vi "model thread map--fgv.vi"(2 "operation":enum16{"Reset", "Insert", "Remove", "find"}(ring), 5 "model name in":string, 7 "model number in":i32, 9 "thread number In":i32, 11 "error in (no error)":errorcluster) -> (4 "Map":map{string, i32}(c390), 6 "model name out":string, 8 "model number out":i32, 10 "thread number out":i32, 15 "error out":errorcluster)   [LabVIEW 2022 SP3]
uses:
  <vilib>/Utility/error.llb/Error Cluster From Error Code.vi
  <vilib>/ErrorRing/Error Ring.xnode
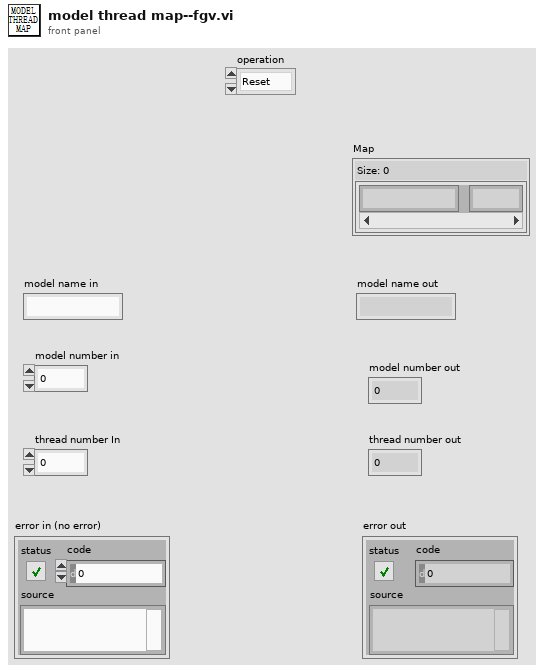
[diagram p1: front panel]
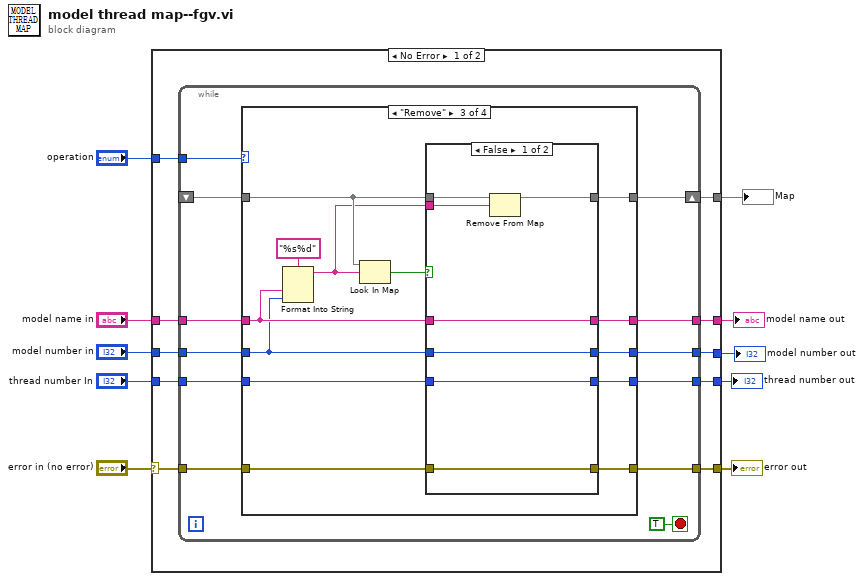
[diagram p0: block diagram]
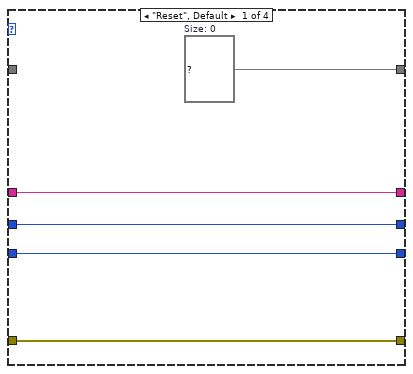
[diagram p2: hidden frame]
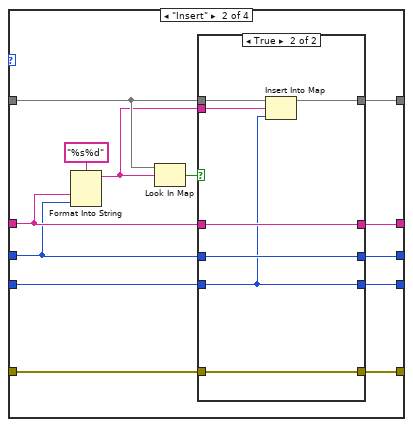
[diagram p3: hidden frame]
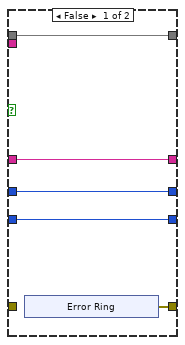
[diagram p4: hidden frame]
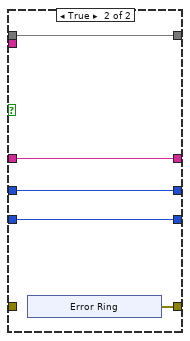
[diagram p5: hidden frame]
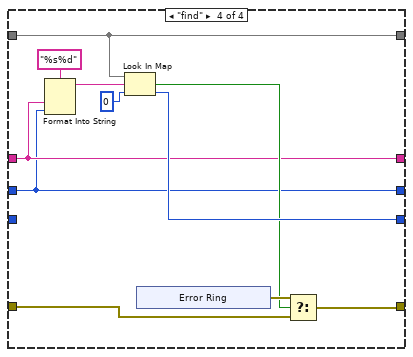
[diagram p6: hidden frame]
diagram:
  n1 = case shown="No Error" "error in (no error)" {
    selector: "error in (no error)" -> [w15 w117]
    tunnel: "operation" -> [w20 _]
    tunnel: "model name in" -> [w19 w116]
    tunnel: "model number in" -> [w18 w115]
    tunnel: [w16 w117] -> w6
    tunnel: "thread number In" -> [w17 w114]
    tunnel: [w14 w114] -> w4
    tunnel: [w13 _] -> w3
    tunnel: [w12 w116] -> w2
    tunnel: [w11 w115] -> w1
    frame No Error {
      n2 = while {
        shift-right: [w30] -> w13
        shift-left: _ -> [w29]
        tunnel: w20 -> [w32]
        tunnel: w19 -> [w28]
        tunnel: w18 -> [w27]
        tunnel: w17 -> [w26]
        tunnel: [w25] -> w16
        tunnel: w15 -> [w24]
        tunnel: [w23] -> w14
        tunnel: [w22] -> w12
        tunnel: [w21] -> w11
        stop <- TRUE stop-if-true
        n3 = case shown="\"Remove\"" w32 {
          tunnel: [w37 w47 w77 w106] -> w30
          tunnel: w29 -> [_ w48 w78 w106]
          tunnel: w28 -> [w35 w42 w73 w99]
          tunnel: w27 -> [w34 w40 w72 w98]
          tunnel: w26 -> [w33 w45 w71 _]
          tunnel: [w36 w44 w75 w104] -> w25
          tunnel: w24 -> [w36 w43 w74 w100]
          tunnel: [w33 w38 w68 w103] -> w23
          tunnel: [w35 w41 w70 w99] -> w22
          tunnel: [w34 w39 w69 w98] -> w21
          frame "Reset", Default {
            w37 = map{string, i32} {}  # Size: 0
          }
          frame "Insert" {
            n4 = Format Into String(format string="%s%d", w42, w40) -> (resulting string=w46:string)  [unwired: 2 in, 1 out]
            n5 = Look In Map(map=w48, key=w46) -> (key not found?=w49:bool)  [unwired: 1 in, 1 out]
            n6 = case shown="True" w49 {
              tunnel: w48 -> [w55 w67]
              tunnel: [w55 w66] -> w47
              tunnel: w46 -> [_ w65]
              tunnel: w45 -> [w51 w61]
              tunnel: [w54 w64] -> w44
              tunnel: w43 -> [_ w64]
              tunnel: w42 -> [w53 w63]
              tunnel: [w53 w63] -> w41
              tunnel: w40 -> [w52 w62]
              tunnel: [w52 w62] -> w39
              tunnel: [w51 w61] -> w38
              frame False {
                n7 = xnode "Error Ring"() -> ("error out"=w54:errorcluster)
              }
              frame True {
                n8 = Insert Into Map(map in=w67, key=w65, value=w61) -> (map out=w66:map{string, i32})  [unwired: 2 out]
              }
            }
          }
          frame "Remove" {
            n9 = Format Into String(format string="%s%d", w73, w72) -> (resulting string=w76:string)  [unwired: 2 in, 1 out]
            n10 = Look In Map(map=w78, key=w76) -> (key not found?=w79:bool)  [unwired: 1 in, 1 out]
            n11 = case shown="False" w79 {
              tunnel: w78 -> [w87 w91]
              tunnel: [w86 w91] -> w77
              tunnel: w76 -> [w85 _]
              tunnel: [w84 w92] -> w75
              tunnel: w74 -> [w84 _]
              tunnel: w73 -> [w83 w90]
              tunnel: w72 -> [w82 w89]
              tunnel: w71 -> [w81 w88]
              tunnel: [w83 w90] -> w70
              tunnel: [w82 w89] -> w69
              tunnel: [w81 w88] -> w68
              frame False {
                n12 = Remove From Map(10:w85, 11:w87) -> (3:w86:map{string, i32})  [unwired: 2 out]
              }
              frame True {
                n13 = xnode "Error Ring"() -> ("error out"=w92:errorcluster)
              }
            }
          }
          frame "find" {
            n14 = Format Into String(format string="%s%d", w99, w98) -> (resulting string=w107:string)  [unwired: 2 in, 1 out]
            n15 = Look In Map(map=w106, key=w107, default value=0) -> (key not found?=w101:bool, value=w103:i32)
            n16 = xnode "Error Ring"() -> ("error out"=w102:errorcluster)
            n17 = Select(t=w102, s=w101, f=w100) -> (s? t:f=w104:errorcluster)
          }
        }
      }
    }
    frame Error {
    }
  }
  "error out" <- w6
  "thread number out" <- w4
  "Map" <- w3
  "model name out" <- w2
  "model number out" <- w1
